vi "Initialise Textures.vi"(8 "error in (no error)":errorcluster, 10 "Renderer":u32, 11 "Ship in":refnum<class "Ship.lvclass">) -> (0 "error out":errorcluster, 3 "Ship out":refnum<class "Ship.lvclass">)   [LabVIEW 2021, in "Ship.lvclass"]
uses:
  Ship.lvclass
  C:/dev/LabVIEW/LabMelee/Source/Application Specific/Element/Element.lvclass
  Ship.lvclass/Ship.ctl
  Element/Element.lvclass/Element.ctl
  Element/Element.lvclass
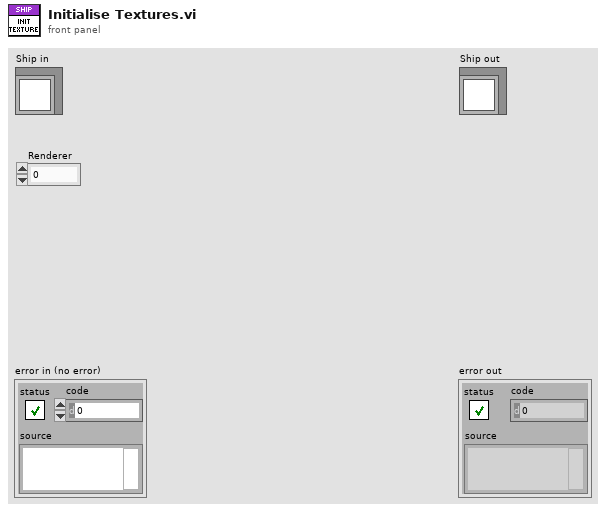
[diagram p1: front panel]
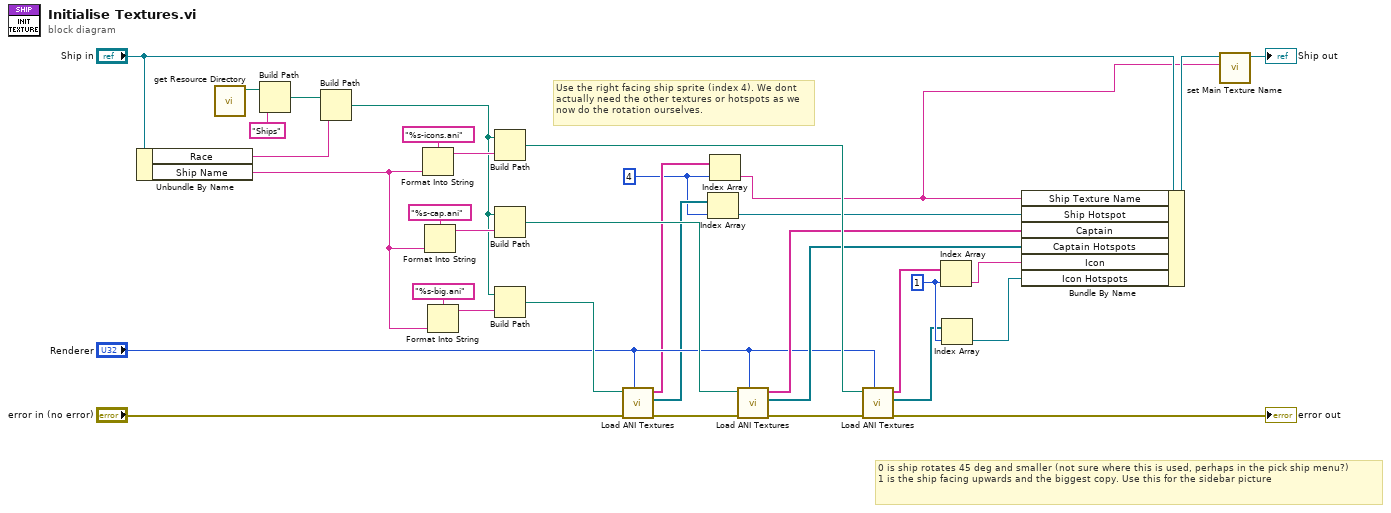
[diagram p0: block diagram]
diagram:
  w4 = 4 ("index")
  w25 = 1 ("index")
  # "Use the right facing ship sprite (index 4). We dont actually need the other textures or hotspots as we now do the rotation ourselves."
  # "0 is ship rotates 45 deg and smaller (not sure where this is used, perhaps in the pick ship menu?)\n1 is the ship facing upwards and the biggest copy. Use this for the sidebar picture"
  n1 = Unbundle By Name("Ship in") -> ("Race"=w19:string, "Ship Name"=w10:string)
  n2 = call "get Resource Directory.vi"() -> ("Resource Directory"=w31:path)  [unwired: 11 in]
  n3 = Build Path(base path=w31, name or relative path="Ships") -> (appended path=w29:path)
  n4 = Build Path(base path=w29, name or relative path=w19) -> (appended path=w11:path)
  n5 = Format Into String(format string="%s-icons.ani", w10) -> (resulting string=w27:string)  [unwired: 2 in, 1 out]
  n6 = Format Into String(format string="%s-cap.ani", w10) -> (resulting string=w33:string)  [unwired: 2 in, 1 out]
  n7 = Format Into String(format string="%s-big.ani", w10) -> (resulting string=w34:string)  [unwired: 2 in, 1 out]
  n8 = Build Path(base path=w11, name or relative path=w27) -> (appended path=w20:path)
  n9 = Build Path(base path=w11, name or relative path=w33) -> (appended path=w21:path)
  n10 = Build Path(base path=w11, name or relative path=w34) -> (appended path=w22:path)
  n11 = call "Load ANI Textures.vi"("Renderer"="Renderer", "error in (no error)"="error in (no error)", "Path"=w22) -> ("error out"=w8:errorcluster, "Hotspots"=w6:refnum<class "Vector 2D.lvclass">[], "Names"=w7:string[])  [unwired: 6 in]
  n12 = Index Array(array=w6, index=w4) -> (element=w5:refnum<class "Vector 2D.lvclass">)
  n13 = Index Array(array=w7, index=w4) -> (element=w1:string)
  n14 = call "Load ANI Textures.vi"("Renderer"="Renderer", "error in (no error)"=w8, "Path"=w21) -> ("error out"=w28:errorcluster, "Hotspots"=w14:refnum<class "Vector 2D.lvclass">[], "Names"=w15:string[])  [unwired: 6 in]
  n15 = call "Load ANI Textures.vi"("Renderer"="Renderer", "error in (no error)"=w28, "Path"=w20) -> ("error out"=→"error out":errorcluster, "Hotspots"=w12:refnum<class "Vector 2D.lvclass">[], "Names"=w13:string[])  [unwired: 6 in]
  n16 = Index Array(array=w13, index=w25) -> (element=w23:string)
  n17 = Index Array(array=w12, index=w25) -> (element=w24:refnum<class "Vector 2D.lvclass">)
  n18 = Bundle By Name(cluster="Ship in", "Ship Texture Name"=w1, "Ship Hotspot"=w5, "Captain"=w15, "Captain Hotspots"=w14, "Icon"=w23, "Icon Hotspots"=w24) -> (w3:refnum<class "Ship.lvclass">)
  n19 = call "set Main Texture Name.vi"("Main Texture Name"=w1, "Element in"=w3) -> ("Element out"=→"Ship out":refnum<class "Ship.lvclass">)  [unwired: 9 in]
